vi "ReadSIAM-Ring.vi"() -> ()   [LabVIEW 2011]
panel:
  in  "Motor-Ticket-Konstants":u32[](array[numeric])=[544, 545, 546, 547, 548] format="%.0x"
  in  "ResolutionBits-Table":u8[][](array[numeric])=[[24, 20, 8, 8], [24, 20, 8, 8], [24, 20, 8, 8], [24, 20, 8, 8], [24, 20, 8, 8]]
  in  "Type":u16(ring) items=["acceleration", "velocity", "position", "offset"]
  in  "Motor":T1(ring)
  in  "Tickets":u16(ring) items=["stdout"=512, "framecountdown"=515, "x"=528, "y"=529, "z"=530, "objective-changer"=531, "maindichro"=532, "Trans-motor5"=533, "FRET-motor6"=534, "SI-motor7"=535, "Galvo0"=544, "Galvo1"=545, "x-Galvo"=546, "y-Galvo"=547, "z-TMSI"=548]
  out "Descriptions":cluster{u32, "ValueText":string}[](array[cluster])=[{17305600, "ValueText"="read status of x-motor, 0=ON_AND_NOT_INIT, 1=ON_AND_INIT, 3=offandinit"}, {17760263, "ValueText"="init x-motor, needs some seconds"}, {16781312, "ValueText"="read x-Motor absolute position in uSteps"}, {16777217, "ValueText"="x-Motor write absolute position in uSteps"}, {16842753, "ValueText"="x-Motor write relative position in uSteps"}, {18354176, "ValueText"="read status of y-motor, 0=ON_AND_NOT_INIT, 1=ON_AND_INIT, 3=offandinit"}, {18808839, "ValueText"="init y-motor, needs some seconds"}, {17829888, "ValueText"="read y-Motor absolute position in uSteps"}, {17825793, "ValueText"="y-Motor write absolute position in uSteps"}, {17891329, "ValueText"="y-Motor write relative position in uSteps"}, {19402752, "ValueText"="read status of z-motor, 0=ON_AND_NOT_INIT, 1=ON_AND_INIT, 3=offandinit"}, {19857415, "ValueText"="init z-motor, needs some seconds"}, {19857423, "ValueText"="stop z-motor, go out of closed loop"}, {19857422, "ValueText"="start z-motor, go into closed loop"}, {18878464, "ValueText"="read z-Motor absolute position in uSteps"}, {18874369, "ValueText"="z-Motor write absolute position in uSteps"}, {18939905, "ValueText"="z-Motor write relative position in uSteps"}, {4027514895, "ValueText"="end without ticket"}, {4027518991, "ValueText"="end with ticket"}, {218107904, "ValueText"="IO-read_bank0"}, {218103809, "ValueText"="IO-write_bank0"}, {219156480, "ValueText"="IO-read_bank1"}, {219152385, "ValueText"="IO-write_bank1"}, {218365953, "ValueText"="next bank0 with highres delay no other IO-write until IO done"}, {218365955, "ValueText"="next bank0 with highres delay, value from variable"}, {3289124864, "ValueText"="read background-measured 100MHz ticks between 256 camclocks"}, {3289120770, "ValueText"="store background-measured 100MHz ticks between 256 camclocks to var"}, {3289190400, "ValueText"="read background-measured 100MHz ticks between rizing cam and 10us"}, {3288989697, "ValueText"="set delay in 100MHz ticks to avoid small result, avoid trigger problems, 100"}, {3289055233, "ValueText"="set future 10µs cycels to calculate modulo"}, {3289055235, "ValueText"="set future 10µs cycels from variable# to calculate modulo"}, {3289317386, "ValueText"="do the modulo calculation, after that the result registers are valid"}, {3289251842, "ValueText"="store modulo result in user variable n"}, {4060086278, "ValueText"="ad value to variable"}, {4060090368, "ValueText"="read variable n"}, {4060086273, "ValueText"="set variable n"}, {4060086276, "ValueText"="copy variable m to n"}, {4043374945, "ValueText"="decrement var and branch (0=same line) if equal, I32"}, {4043375201, "ValueText"="decrement var and branch (0=same line) if greater or equal, I32"}, {4043379297, "ValueText"="decrement and branch (0=same line) if greater or equal"}, {4043375457, "ValueText"="decrement and branch (0=same line) if smaller, I32"}, {4043375473, "ValueText"="increment and branch (0=same line) if smaller, I32"}, {102760689, "ValueText"="x-Galvo,data order o,pos,vel,acc"}, {103809265, "ValueText"="y-Galvo,o,pos,vel,acc"}, {104857841, "ValueText"="z-focus,o,pos,vel,acc"}, {102760513, "ValueText"="x-Galvo,pos in data1"}, {103809089, "ValueText"="y-Galvo,pos in data1"}, {104857665, "ValueText"="z-focus,pos in data1"}, {102764609, "ValueText"="x-Galvo,pos in data1, ticket"}, {103813185, "ValueText"="y-Galvo,pos in data1, ticket"}, {104861761, "ValueText"="z-focus,pos in data1, ticket"}, {102764608, "ValueText"="read x-Galvo-pos,ticket"}, {103813184, "ValueText"="read y-Galvo-pos,ticket"}, {104861760, "ValueText"="read z-Focus-pos,ticket"}, {102760515, "ValueText"="set x-Galvo-pos from variable"}, {103809091, "ValueText"="set y-Galvo-pos from variable"}, {104857667, "ValueText"="set z-Focus-pos from variable"}] {"?" format="%.0x"}
  in  "command":u32(ring)=4027514895 format="%x" items=["end_no_ticket"=4027514895, "end_ticket"=4027518991, "NoOp"=4026531840, "Read ticks"=4026535936, "Read ticks to var"=4026535938, "Read IP"=4043313152, "Read IP into var"=4043313154, "Set IP from var"=4043309059, "Set IP from var, relative"=4043313155, "branchRel_if_equal"=4043374849, "decrement_branchRel_if_equal"=4043374945, "decrement_branchRel_if_greaterequal"=4043375201, "decrement_branchRel_if_greaterequal_withTicket"=4043379297, "decrement_branchRel_if_smaller"=4043375457, "increment_branchRel_if_smaller"=4043375473, "readVar"=4060090368, "writeVar"=4060086273, "copyVar0_from_var1"=4060086275, "math_addToVariable"=4076863488, "math_addVToVariable"=4076863489, "math_subToVariable"=4076863490, "math_subVToVariable"=4076863491, "math_multToVariable"=4076863492, "math_multvToVariable"=4076863493, "math_divideToVariable"=4076863494, "math_divideVToVariable"=4076863495, "math_modToVariable"=4076863496, "math_modVToVariable"=4076863497, "logic_and"=4093640704, "logic_or"=4093640706, "logic_xor"=4093640708, "bitshift"=4093640712, "I2C-write"=335544337, "I2C-read"=335548433, "Cam-SPI-write"=3254779905, "UART0-VC-Baud-write"=469958673, "UART0-VC-Baud-read"=469962768, "UART0-VC-write"=469762065, "UART0-VC-write-Var"=469762067, "UART0-VC-read-availabe-bytes-to-var"=470355970, "UART0-VC-read-availabe-bytes"=470355984, "UART0-VC-read-skip-bytes"=469831681, "UART0-VC-read"=469766160, "UART0-VC-read-Var"=469766162, "UART1-TSM-Baud-write"=486735889, "UART1-TSM-Baud-read"=486739984, "UART1-TSM-write"=486539281, "UART1-TSM-write-Var"=486539283, "UART1-TSM-read-availabe-bytes-to-var"=487133186, "UART1-TSM-read-availabe-bytes"=487133200, "UART1-TSM-read-skip-bytes"=486604801, "UART1-TSM-read-skip-bytes"=486608897, "UART1-TSM-read"=486543376, "UART1-TSM-read-Var"=486543378, "UART2-Laser-Baud-write"=503513105, "UART2-Baud-read"=503517200, "UART2-write"=503316497, "UART2-write-Var"=503316499, "UART2-read-availabe-bytes-to-var"=503910402, "UART2-read-availabe-bytes"=503910416, "UART2-read-skip-bytes"=503386113, "UART2-read"=503320592, "UART2-read-Var"=503320594, "UART3-Baud-write"=520290321, "UART3-Baud-read"=520294416, "UART3-write"=520093713, "UART3-write-Var"=520093715, "UART3-read-availabe-bytes-to-var"=520687618, "UART3-read-availabe-bytes"=520687632, "UART3-read-skip-bytes"=520163329, "UART3-read"=520097808, "UART3-read-Var"=520097810, "IO-read_bank0"=3489665024, "IO-write_bank0"=3489660929, "IO-read_bank1"=3506442240, "IO-write_bank1"=3506438145, "DA0-0_LED365"=2684354561, "DA0-1_LED385"=2685403137, "DA0-2_LED440"=2686451713, "DA0-3_LED470"=2687500289, "DA0-4_LED510"=2688548865, "DA0-5_LED550"=2689597441, "DA0-6_LED590"=2690646017, "DA0-7_LED640"=2691694593, "DA1-0_LED-R"=2701131777, "DA1-1_LED-G"=2702180353, "DA1-2_LED-B"=2703228929, "DA1-3_LED-AF"=2704277505, "DA1-4"=2705326081, "DA1-5"=2706374657, "DA1-6"=2707423233, "DA1-7"=2708471809, "DA2-Laser0"=2717908993, "DA2-Laser1"=2718957569, "DA2-Laser2"=2720006145, "DA2-Laser3"=2721054721, "DA2-Laser4"=2722103297, "Analog-read_AD0-0"=2818576384, "Analog-read-store_AD0-0"=2818572290, "AF-Register-transfer r/w"=2835349505, "AF-Register-read"=2835353600, "AF-Register-read-to-var"=2835353602, "AF-Transfer-from-var"=2835349507, "IO-delay_bank0"=3489923073, "IO-delay_bank0_fromVar"=3489923075, "read_cam_clock"=3289124864, "store_cam_clock"=3289120770, "read_cam_phase"=3289190400, "store_cam_phase"=3289186306, "store_cam_phase-t"=3289190402, "r_cam1_NHS"=3254980608, "w_cam1_NHS"=3254976513, "r_cam1_NVS"=3255046144, "w_cam1_NVS"=3255042049, "r_cam1_npx"=3255111680, "w_cam1_npx"=3255107585, "r_cam1_npy"=3255177216, "w_cam1_npy"=3255173121, "r_cam1_xhswait"=3255439360, "w_cam1_xhswait"=3255435265, "r_cam1_xvs_wait"=3255504896, "w_cam1_xvs_wait"=3255500801, "r_cam1_framcounter"=3255570432, "r_cam1_line"=3255635968, "r_cam1_xhs-counter"=3255701504, "r_cam2_NHS"=3271757824, "w_cam2_NHS"=3271753729, "r_cam2_NVS"=3271823360, "w_cam2_NVS"=3271819265, "r_cam2_npx"=3271888896, "w_cam2_npx"=3271884801, "r_cam2_npy"=3271954432, "w_cam2_npy"=3271950337, "r_cam2_xvs_wait"=3272282112, "w_cam2_xvs_wait"=3272278017, "r_cam2_framcounter"=3272347648, "r_cam2_line"=3272413184, "r_cam2_xhs-counter"=3272478720, "start TMSI"=102694919, "set_1Galvo"=101712113, "set_x-Galvo"=102760689, "set_y-Galvo"=103809265, "set_z-Fokus"=104857841, "set_1Galvo_position-only"=101711937, "set_x-Galvo_position-only"=102760513, "set_y-Galvo_position-only"=103809089, "set_z-Fokus_position-only"=104857665, "set_x-Galvo_position-only_ticket"=102764609, "set_y-Galvo_position-only_ticket"=103813185, "set_z-Fokus_position-only_ticket"=104861761, "set_1Galvo_relativ-only"=101712001, "set_x-Galvo_relativ-only"=102760577, "set_y-Galvo_relativ-only"=103809153, "set_z-Fokus_relativ-only"=104857729, "set_1Galvo_speed-only"=101711905, "set_x-Galvo_speed-only"=102760481, "set_y-Galvo_speed-only"=103809057, "set_z-Fokus_speed-only"=104857633, "set_1Galvo_acc-only"=101711889, "set_x-Galvo_acc-only"=102760465, "set_y-Galvo_acc-only"=103809041, "set_z-Fokus_acc-only"=104857617, "read_1Galvo_ticket"=101716032, "read_x-Galvo_ticket"=102764608, "read_y-Galvo_ticket"=103813184, "read_z-Focus_ticket"=104861760, "x-Galvo_pos_fromVar"=102760515, "y-Galvo_pos_fromVar"=103809091, "z-Focus_pos_fromVar"=104857667, "Servo0"=67108865, "Servo0-enable"=68091911, "Servo0-disable"=68091919, "Servo1"=68157441, "Servo1-enable"=69140487, "Servo1-disable"=69140495, "Servo2-enable"=70189063, "Servo2"=69206017, "Servo3-enable"=71237639, "Servo3"=70254593, "x-ssi-init"=202309639, "x-ssi-disable"=202309647, "x-ssi-Bits"=201523201, "x-ssi-Read"=201330688, "x-ssi-ReadToVar"=201326594, "x-ssi-ReadToVar-ticket"=201330690, "y-ssi-init"=203358215, "y-ssi-disable"=203358223, "y-ssi-Bits"=202571777, "y-ssi-Read"=202379264, "y-ssi-ReadToVar"=202375170, "y-ssi-ReadToVat-ticket"=202379266]
  in  "String":string="/* This is a idea of a program readable SAM command description, perhaps we could get that from the board? */\n/* 2021.12.07 new version for ImgProc1-FPGA, rename to RIC!*/\n/* Only the DeviceID+Command and Data structure is explained, communication commands are quite fixed! */\n/* all Values are 32bit, usually signed integer */\n/* there is 8x32bits, a relative time, a command, 5 values (data0 to data4), and data5 for the return ticket */\n/* up to ~14 commands are possible with time delay=0 */\n/* last 4 command bit: 0=read, 1=write, 2=store to var, 3=load from var\" */\n/* xxxx1xxx command ist with ticket return */\n/* TMSI data alignment change after Rev 3 (bug between 3.1-3.8) */\n/* raw commands changed 2018 xxxxxx10, obsolete?, raw read now fpga does not wait */\n/* \\\\till-server\\work\\Projekte allgemein\\Platinen\\SAM-Boards\\SAM2 Board v1.0 Paraxent\\SAM2_Board_all_opcodes.xlsx  */\n\n/*Slow motors via Linux: Does not exist any more; use UART raw! */\n/* fast 10µs commands */\n/*program commands */\ncommand=\"OxF00F000F\" name=\"end_no_ticket\" description=\"end without ticket\"\ncommand=\"OxF00F100F\" name=\"end_ticket\" description=\"end with ticket\" data5-description=\"return-ticket\"\ncommand=\"0xF0000000\" name=\"NoOp\" description=\"Nix, eigentlich...tickcounter\"\n/* 10µs tick counter */\ncommand=\"0xF0001000\" name=\"Read ticks\" description=\"read 10µs counter\"\ncommand=\"0xF0001002\" name=\"Read ticks to var\" description=\"store 10µs to variable\" data0-description=\"variable#\"\n/* Instruction pointer manipulation = jumps */\ncommand=\"0xF1001000\" name=\"Read IP\" description=\"read Instruction pointer\" data5-description=\"return-ticket\"\ncommand=\"0xF1001002\" name=\"Read IP into var\" description=\"read Instruction pointer into variable\" data0-type=U32 data0-description=\"Var#\" data5-description=\"return-ticket\"\ncommand=\"0xF1000003\" name=\"Set IP from var\" description=\"set Instruction pointer from variable\" data0-type=U32 data0-description=\"Var#\"\ncommand=\"0xF1001003\" name=\"Set IP from var, relative\" description=\"set Instruction pointer from variable, relative to actual pointer\" data0-type=U32 data0-description=\"Var# with signed I32\" data5-description=\"return-ticket\"\n/* branch */\ncommand=\"0xF1010101\" name=\"branchRel_if_equal\" description=\"branch (0=same line) if var# equal konstant, I32\" data0-descrition=\"relative jump lines 0=same line\" data0-type=I32 data1-description=\"variable# (0-FF)\" data2-description=\"compare value\" data2-type=I32 \ncommand=\"0xF1010161\" name=\"decrement_branchRel_if_equal\" description=\"decrement var and branch (0=same line) if equal, I32\" data0-descrition=\"relative jump lines 0=same line\" data0-type=I32 data1-description=\"variable# (0-??)\" data2-description=\"compare value\" data2-type=I32 \ncommand=\"0xF1010261\" name=\"decrement_branchRel_if_greaterequal\" description=\"decrement var and branch (0=same line) if greater or equal, I32\" data0-descrition=\"relative jump lines 0=same line\" data0-type=I32 data1-description=\"variable# (0-FF)\" data2-description=\"compare value\" data2-type=I32 \ncommand=\"0xF1011261\" name=\"decrement_branchRel_if_greaterequal_withTicket\" description=\"decrement and branch (0=same line) if greater or equal\" data0-descrition=\"relative jump lines\" data0-type=I32 data1-description=\"variable# (0-FF)\" data2-description=\"compare value\" data1-type=I32 data5-description=\"return-ticket\" \ncommand=\"0xF1010361\" name=\"decrement_branchRel_if_smaller\" description=\"decrement and branch (0=same line) if smaller, I32\" data0-descrition=\"relative jump lines 0=same line\" data0-type=I32 data1-description=\"variable# (0-FF)\" data2-description=\"compare value\" data2-type=I32 \ncommand=\"0xF1010371\" name=\"increment_branchRel_if_smaller\" description=\"increment and branch (0=same line) if smaller, I32\" data0-descrition=\"relative jump lines 0=same line\" data0-type=I32 data1-description=\"variable# (0-FF)\" data2-description=\"compare value\" data2-type=I32 \n/* variables */\ncommand=\"0xF2001000\" name=\"readVar\" description=\"read variable n\" data0-description=\"variable# (0-??), also registers!\" data5-description=\"return-ticket\"\ncommand=\"0xF2000001\" name=\"writeVar\" description=\"set variable n\" data0-description=\"variable# (0-??)\" data1-description=\"value\" data1-type=I32\ncommand=\"0xF2000003\" name=\"copyVar0_from_var1\" description=\"copy var data1 to var data0\" data0-description=\"traget variable# (0-FF)\" data0-type=U8 data1-description=\"source Variable#\" data1-type=U8\n/* math, result always in data0*/\ncommand=\"0xF3000000\" name=\"math_addToVariable\" description=\"add variable0 and value\" data0-description=\"variable#, result\" data1-description=\"valueI32\"\ncommand=\"0xF3000001\" name=\"math_addVToVariable\" description=\"add variable1 to variable0\" data0-description=\"variable#, result\" data1-description=\"variable#\"\ncommand=\"0xF3000002\" name=\"math_subToVariable\" description=\"sub value from variable0\" data0-description=\"variable#, result\" data1-description=\"valueI32\"\ncommand=\"0xF3000003\" name=\"math_subVToVariable\" description=\"sub variable1 from variable0\" data0-description=\"variable0#, result\" data1-description=\"variable1#\"\ncommand=\"0xF3000004\" name=\"math_multToVariable\" description=\"multiply variable with value\" data0-description=\"variable#, result\" data1-description=\"valueI32\"\ncommand=\"0xF3000005\" name=\"math_multvToVariable\" description=\"multiply variable0 with variable1\" data0-description=\"variable0, result#\" data1-description=\"variable1#\"\ncommand=\"0xF3000006\" name=\"math_divideToVariable\" description=\"divide variable0 with value\" data0-description=\"variable#, result\" data1-description=\"valueI32\"\ncommand=\"0xF3000007\" name=\"math_divideVToVariable\" description=\"divide variable1 with variable2\" data0-description=\"variable0#, result\" data1-description=\"variable1#\"\ncommand=\"0xF3000008\" name=\"math_modToVariable\" description=\"integer devision rest variable/value\" data0-description=\"variable#, result\" data1-description=\"valueI32\"\ncommand=\"0xF3000009\" name=\"math_modVToVariable\" description=\"integer devision rest variable0/variable1\" data0-description=\"variable0#, result\" data1-description=\"variable1#\"\n/* logics */\ncommand=\"0xF4000000\" name=\"logic_and\" description=\"variable and value\" data0-description=\"variable#\" data1-description=\"valueI32\"\ncommand=\"0xF4000002\" name=\"logic_or\" description=\"variable or value\" data0-description=\"variable#\" data1-description=\"valueI32\"\ncommand=\"0xF4000004\" name=\"logic_xor\" description=\"variable exclusiveor value\" data0-description=\"variable#\" data1-description=\"valueI32\"\ncommand=\"0xF4000008\" name=\"bitshift\" description=\"shift bits right = devide 2^n, (do left with mult)\" data0-description=\"variable#\" data1-description=\"valueI32 (0-32?)\"\n/*I2C commands */\ncommand=\"0x14000011\" name=\"I2C-write\" description=\"I2C-write\" data0-descrition=AABBCCDD: AA=i2c-addr Tango0x72, CC send bytes, DD response bytes\", data1-description=\"send byts\", data2-description=\"send bytes\", data5-description=\"return ticket\" \ncommand=\"0x14001011\" name=\"I2C-read\" description=\"I2C-read\" data0-descrition=AABBCCDD: AA=i2c-addr Tango0x72, CC send bytes, DD response bytes\", data1-description=\"send byts\", data2-description=\"send bytes\", data5-description=\"return ticket\" \n/*SPI-Camera commands */\ncommand=\"0xC2000001\" name=\"Cam-SPI-write\" description=\"Cam-Write\" data0-descrition=\"0000writebytes(1-F)00\" data1-description=\"data bytes 1,2,3,4\" data2-description=\"data bytes 5,6,7,8\" data3-description=\"data bytes 9,10,11,12\" data4-description=\"data bytes 13,14,15,16\"\n\n/* UART raw commands */\ncommand=\"0x1C030011\" name=\"UART0-VC-Baud-write\" description=\"DCC22-Baud-write\" data0-descrition=\"9600:0xD, 57600: 0x1001, default>115200: 0x1002\" \ncommand=\"0x1C031010\" name=\"UART0-VC-Baud-read\" description=\"DCC22-Baud-read 9600:0xD, 57600: 0x1001, >115200: 0x1002\" \ncommand=\"0x1C000011\" name=\"UART0-VC-write\" description=\"DCC22-write\" data0-descrition=\"0000writebytes(1-F)00\" data1-description=\"data bytes 1,2,3,4\" data2-description=\"data bytes 5,6,7,8\" data3-description=\"data bytes 9,10,11,12\" data4-description=\"data bytes 13,14,15,16\"\ncommand=\"0x1C000013\" name=\"UART0-VC-write-Var\" description=\"DCC22-write from Var\" data0-descrition=\"0000writebytes(1-4)00, big endian\" data1-description=\"var#\"\ncommand=\"0x1C091002\" name=\"UART0-VC-read-availabe-bytes-to-var\" description=\"DCC22-read available bytes, fifo is 1024 long\" data0-descrition=\"var#\" data5-description=\"return ticket\" \ncommand=\"0x1C091010\" name=\"UART0-VC-read-availabe-bytes\" description=\"DCC22-read available bytes, fifo is 1024 long\" data5-description=\"return ticket\" \ncommand=\"0x1C011001\" name=\"UART0-VC-read-skip-bytes\" description=\"DCC22-read-fifo skip bytes\" data0-descrition=\"number of bytes, should not exced available bytes\" data5-description=\"return ticket\" \ncommand=\"0x1C001010\" name=\"UART0-VC-read\" description=\"DCC22-read, big endian packed in U32\" data0-descrition=\"bytes (1-4), FFFFFFFF=all(but ticket not working)\" data5-description=\"return ticket\" \ncommand=\"0x1C001012\" name=\"UART0-VC-read-Var\" description=\"DCC22-read to Var, big endian\" data0-descrition=\"bytes(01-04)\" data1-description=\"var#\" data5-description=\"return ticket\" \ncommand=\"0x1D030011\" name=\"UART1-TSM-Baud-write\" description=\"TSM-Baud-read 9600:0xD, default>57600: 0x1001, 115200: 0x1002\" \ncommand=\"0x1D031010\" name=\"UART1-TSM-Baud-read\" description=\"TSM-Baud-read 9600:0xD, >57600: 0x1001, 115200: 0x1002\" \ncommand=\"0x1D000011\" name=\"UART1-TSM-write\" description=\"TSM-write\" data0-descrition=\"0000writebytes(1-F)00\" data1-description=\"data bytes 1,2,3,4\" data2-description=\"data bytes 5,6,7,8\" data3-description=\"data bytes 9,10,11,12\" data4-description=\"data bytes 13,14,15,16\"\ncommand=\"0x1D000013\" name=\"UART1-TSM-write-Var\" description=\"TSM-write from Var\" data0-descrition=\"0000writebytes(1-4)00, big endian\" data1-description=\"var#\"\ncommand=\"0x1D091002\" name=\"UART1-TSM-read-availabe-bytes-to-var\" description=\"TSM-read available bytes, fifo is 1024 long\" data0-descrition=\"var#\" data5-description=\"return ticket\" \ncommand=\"0x1D091010\" name=\"UART1-TSM-read-availabe-bytes\" description=\"TSM-read available bytes, fifo is 1024 long\" data5-description=\"return ticket\" \ncommand=\"0x1D010001\" name=\"UART1-TSM-read-skip-bytes\" description=\"TSM-read-fifo skip bytes\" data0-descrition=\"number of bytes, should not exced available bytes, gibts nicht bei sam1\"\ncommand=\"0x1D011001\" name=\"UART1-TSM-read-skip-bytes\" description=\"TSM-read-fifo skip bytes\" data0-descrition=\"number of bytes, should not exced available bytes\" data5-description=\"return ticket\" \ncommand=\"0x1D001010\" name=\"UART1-TSM-read\" description=\"TSM-read, big endian packed in U32\" data0-descrition=\"bytes (1-4), FFFFFFFF=all(old? but ticket not working)\" data5-description=\"return ticket\" \ncommand=\"0x1D001012\" name=\"UART1-TSM-read-Var\" description=\"TSM-read to Var, big endian\" data0-descrition=\"bytes(01-04)\" data1-description=\"var#\" data5-description=\"return ticket\" \ncommand=\"0x1E030011\" name=\"UART2-Laser-Baud-write\" description=\"Laser-Baud-write\" data0-descrition=\"9600:0xD, 57600: 0x1001, default >115200: 0x1002\" \ncommand=\"0x1E031010\" name=\"UART2-Baud-read\" description=\"Laser-Baud-read 9600:0xD, 57600: 0x1001, 115200: 0x1002\" \ncommand=\"0x1E000011\" name=\"UART2-write\" description=\"Laser-write\" data0-descrition=\"0000writebytes(1-F)00\" data1-description=\"data bytes 1,2,3,4\" data2-description=\"data bytes 5,6,7,8\" data3-description=\"data bytes 9,10,11,12\" data4-description=\"data bytes 13,14,15,16\"\ncommand=\"0x1E000013\" name=\"UART2-write-Var\" description=\"Laser-write from Var\" data0-descrition=\"0000writebytes(1-4)00, big endian\" data1-description=\"var#\"\ncommand=\"0x1E091002\" name=\"UART2-read-availabe-bytes-to-var\" description=\"Laser-read available bytes, fifo is 1024 long\" data0-descrition=\"var#\" data5-description=\"return ticket\" \ncommand=\"0x1E091010\" name=\"UART2-read-availabe-bytes\" description=\"Laser-read available bytes, fifo is 1024 long\" data5-description=\"return ticket\" \ncommand=\"0x1E011001\" name=\"UART2-read-skip-bytes\" description=\"Laser-read-fifo skip bytes\" data0-descrition=\"number of bytes, should not exced available bytes\" data5-description=\"return ticket\" \ncommand=\"0x1E001010\" name=\"UART2-read\" description=\"Laser-read, big endian packed in U32\" data0-descrition=\"bytes (1-4), FFFFFFFF=all(but ticket not working)\" data5-description=\"return ticket\" \ncommand=\"0x1E001012\" name=\"UART2-read-Var\" description=\"Laser-read to Var, big endian\" data0-descrition=\"bytes(01-04)\" data1-description=\"var#\" data5-description=\"return ticket\" \ncommand=\"0x1F030011\" name=\"UART3-Baud-write\" description=\"UART3 Baud-write\" data0-descrition=\"9600:0xD, 57600: 0x1001, 115200: 0x1002\" \ncommand=\"0x1F031010\" name=\"UART3-Baud-read\" description=\"uart3-Baud-read 9600:0xD, 57600: 0x1001, 115200: 0x1002-default\" \ncommand=\"0x1F000011\" name=\"UART3-write\" description=\"uart3-write\" data0-descrition=\"0000writebytes(1-F)00\" data1-description=\"data bytes 1,2,3,4\" data2-description=\"data bytes 5,6,7,8\" data3-description=\"data bytes 9,10,11,12\" data4-description=\"data bytes 13,14,15,16\"\ncommand=\"0x1F000013\" name=\"UART3-write-Var\" description=\"uart3-write from Var\" data0-descrition=\"0000writebytes(1-4)00, big endian\" data1-description=\"var#\"\ncommand=\"0x1F091002\" name=\"UART3-read-availabe-bytes-to-var\" description=\"uart3-read available bytes, fifo is 1024 long\" data0-descrition=\"var#\" data5-description=\"return ticket\" \ncommand=\"0x1F091010\" name=\"UART3-read-availabe-bytes\" description=\"uart3-read available bytes, fifo is 1024 long\" data5-description=\"return ticket\" \ncommand=\"0x1F011001\" name=\"UART3-read-skip-bytes\" description=\"uart3-read-fifo skip bytes\" data0-descrition=\"number of bytes, should not exced available bytes\" data5-description=\"return ticket\" \ncommand=\"0x1F001010\" name=\"UART3-read\" description=\"uart3-read, big endian packed in U32\" data0-descrition=\"bytes (1-4), FFFFFFFF=all(but ticket not working), Error E7 if not enaugh data\" data5-description=\"return ticket\" \ncommand=\"0x1F001012\" name=\"UART3-read-Var\" description=\"uart3-read to Var, big endian\" data0-descrition=\"bytes(01-04)\" data1-description=\"var#\" data5-description=\"return ticket\" \n/* Digital IO */\ncommand=\"0xD0001000\" name=\"IO-read_bank0\" description=\"IO-read_bank0\" data0-descrition=\"mask-needed,Bit1=cam0ready,Bit4=TSMx,Bit5=TSMy,Bit7(0x80)=Deckel nicht offen\" data5-description=\"return ticket\" \ncommand=\"0xD0000001\" name=\"IO-write_bank0\" description=\"IO-write_bank0\" data0-descrition=\"mask\" data1-description=\"values 0x1=Cam; 0x800=470nmLED; 0x100000=laser0;1F0 0000 all lasers\"\ncommand=\"0xD1001000\" name=\"IO-read_bank1\" description=\"IO-read_bank1\" data0-descrition=\"mask\" data5-description=\"return ticket\" \ncommand=\"0xD1000001\" name=\"IO-write_bank1\" description=\"IO-write_bank1\" data0-descrition=\"mask\" data1-description=\"values \"\n/* Analog Out */\ncommand=\"0xA0000001\" name=\"DA0-0_LED365\" description=\"DA0-0-write 365\" data0-descrition=\"Analog 0-3,3V\" data0-type=U16\ncommand=\"0xA0100001\" name=\"DA0-1_LED385\" description=\"DA0-1-write 385\" data0-descrition=\"Analog 0-3,3V\" data0-type=U16\ncommand=\"0xA0200001\" name=\"DA0-2_LED440\" description=\"DA0-2-write 440\" data0-descrition=\"Analog 0-3,3V\" data0-type=U16\ncommand=\"0xA0300001\" name=\"DA0-3_LED470\" description=\"DA0-3-write 470\" data0-descrition=\"Analog 0-3,3V\" data0-type=U16\ncommand=\"0xA0400001\" name=\"DA0-4_LED510\" description=\"DA0-4-write 510\" data0-descrition=\"Analog 0-3,3V\" data0-type=U16\ncommand=\"0xA0500001\" name=\"DA0-5_LED550\" description=\"DA0-5-write 5xx\" data0-descrition=\"Analog 0-3,3V\" data0-type=U16\ncommand=\"0xA0600001\" name=\"DA0-6_LED590\" description=\"DA0-6-write 590\" data0-descrition=\"Analog 0-3,3V\" data0-type=U16\ncommand=\"0xA0700001\" name=\"DA0-7_LED640\" description=\"DA0-7-write 640\" data0-descrition=\"Analog 0-3,3V\" data0-type=U16\ncommand=\"0xA1000001\" name=\"DA1-0_LED-R\" description=\"DA1-0-write R\" data0-descrition=\"Analog 0-3,3V\" data0-type=U16\ncommand=\"0xA1100001\" name=\"DA1-1_LED-G\" description=\"DA1-1-write\" data0-descrition=\"Analog 0-3,3V\" data0-type=U16\ncommand=\"0xA1200001\" name=\"DA1-2_LED-B\" description=\"DA1-2-write\" data0-descrition=\"Analog 0-3,3V\" data0-type=U16\ncommand=\"0xA1300001\" name=\"DA1-3_LED-AF\" description=\"DA1-3-write\" data0-descrition=\"Analog 0-3,3V\" data0-type=U16\ncommand=\"0xA1400001\" name=\"DA1-4\" description=\"DA1-4-write\" data0-descrition=\"Analog 0-3,3V\" data0-type=U16\ncommand=\"0xA1500001\" name=\"DA1-5\" description=\"DA1-5-write\" data0-descrition=\"Analog 0-3,3V\" data0-type=U16\ncommand=\"0xA1600001\" name=\"DA1-6\" description=\"DA1-6-write\" data0-descrition=\"Analog 0-3,3V\" data0-type=U16\ncommand=\"0xA1700001\" name=\"DA1-7\" description=\"DA1-7-write\" data0-descrition=\"Analog 0-3,3V\" data0-type=U16\ncommand=\"0xA2000001\" name=\"DA2-Laser0\" description=\"DA2-Laser0-405?write\" data0-descrition=\"Analog 0-65535\" data0-type=U16\ncommand=\"0xA2100001\" name=\"DA2-Laser1\" description=\"DA2-Laser1-488?write\" data0-descrition=\"Analog 0-65535\" data0-type=U16\ncommand=\"0xA2200001\" name=\"DA2-Laser2\" description=\"DA2-Laser2-561?write\" data0-descrition=\"Analog 0-65535\" data0-type=U16\ncommand=\"0xA2300001\" name=\"DA2-Laser3\" description=\"DA2-Laser3-640?write\" data0-descrition=\"Analog 0-65535\" data0-type=U16\ncommand=\"0xA2400001\" name=\"DA2-Laser4\" description=\"DA2-Laser4-extra-write\" data0-descrition=\"Analog 0-65535\" data0-type=U16\n/* Analog in, no hardware available */\ncommand=\"0xA8001000\" name=\"Analog-read_AD0-0\" description=\"AD0-0-read\" data5-descrition=\"ticket\"\ncommand=\"0xA8000002\" name=\"Analog-read-store_AD0-0\" description=\"AD0-0-read\" data0-descrition=\"Variable# (0-FF)\" data0-type=U32\n/*Autofocus SPI communication */\ncommand=\"0xA9000001\" name=\"AF-Register-transfer r/w\" description=\"R/W in AF-Register\" data0-descrition=\"6bit Adresse, 1=write 0=read,0, 24bit Wert bei write; diode0-read:C0000000; diode1-read:C4000000, diode15-read:FC000000, \"\ncommand=\"0xA9001000\" name=\"AF-Register-read\" description=\"Read transferred SPI-register, >2µs later\" data5-descrition=\"ticket\"\ncommand=\"0xA9001002\" name=\"AF-Register-read-to-var\" description=\"Read transferred SPI-register to var, >2µs later\" data0-description=\"Variable#\" data5-descrition=\"ticket\"\ncommand=\"0xA9000003\" name=\"AF-Transfer-from-var\" description=\"var to Transfer SPI-register, not tested\" data0-description=\"Variable#, top 6 bit is adress, 1 write... 24bit values\"\n/* extra command for high resolution delay, take care to not use other IO-write on this bank until the delayed IO is done */\ncommand=\"0xD0040001\" name=\"IO-delay_bank0\" description=\"next bank0 with highres delay no other IO-write until IO done\" data0-descrition=\"delay in 100MHz?\"\ncommand=\"0xD0040003\" name=\"IO-delay_bank0_fromVar\" description=\"next bank0 with highres delay 100MHz, value from variable\" data0-descrition=\"variable#\"\n/* external cam-sync, measure clock, measure phase, do modulo (100MHz-base) */\ncommand=\"0xC40C1000\" name=\"read_cam_clock\" description=\"read background-measured 100MHz ticks between 256 camlineclocks\" data5-description=\"return-ticket\"\ncommand=\"0xC40C0002\" name=\"store_cam_clock\" description=\"store background-measured 100MHz ticks between 256 camlineclocks to var\" data0-description=\"variable#\"\ncommand=\"0xC40D1000\" name=\"read_cam_phase\" description=\"read background-measured 100MHz ticks between rizing camline and last 10us\" data5-description=\"return-ticket\"\ncommand=\"0xC40D0002\" name=\"store_cam_phase\" description=\"store background-measured 100MHz ticks between rizing camline and last 10us to var\" data0-description=\"variable#\"\ncommand=\"0xC40D1002\" name=\"store_cam_phase-t\" description=\"store background-measured 100MHz ticks between rizing camline and last 10us to var\" data0-description=\"variable#\" data5-description=\"return-ticket\"\n/* sensovation camera\ncommand=\"0xC2031000\" name=\"r_cam1_NHS\" description=\"John1 NHS default 964\" data5-description=\"return-ticket\"\ncommand=\"0xC2030001\" name=\"w_cam1_NHS\" description=\"John1 NHS default 964\" data1-description=\"HS divider\"\ncommand=\"0xC2041000\" name=\"r_cam1_NVS\" description=\"John1 NVS default 3730\" data5-description=\"return-ticket\"\ncommand=\"0xC2040001\" name=\"w_cam1_NVS\" description=\"John1 NVS default 3730\" data1-description=\"VS divider=lines\"\ncommand=\"0xC2051000\" name=\"r_cam1_npx\" description=\"John1 x-pixel default 5632\" data5-description=\"return-ticket\"\ncommand=\"0xC2050001\" name=\"w_cam1_npx\" description=\"John1 x-pixel default 5632\" data1-description=\"VS divider=lines\"\ncommand=\"0xC2061000\" name=\"r_cam1_npy\" description=\"John1 y-pixel default 3708 beendet DMA!\" data5-description=\"return-ticket\"\ncommand=\"0xC2060001\" name=\"w_cam1_npy\" description=\"John1 y-pixel default 3708 beendet DMA!\" data1-description=\"VS divider=lines\"\ncommand=\"0xC20A1000\" name=\"r_cam1_xhswait\" description=\"John1 xvs_wait default 100\" data5-description=\"return-ticket\"\ncommand=\"0xC20A0001\" name=\"w_cam1_xhswait\" description=\"John1 xvs_wait default 100\" data1-description=\"xhs_wait\"\ncommand=\"0xC20B1000\" name=\"r_cam1_xvs_wait\" description=\"John1 xvs_wait default 10 war mal für cam1 und2\" data5-description=\"return-ticket\"\ncommand=\"0xC20B0001\" name=\"w_cam1_xvs_wait\" description=\"John1 xvs_wait default 10\" data1-description=\"xvs_wait\"\ncommand=\"0xC20C1000\" name=\"r_cam1_framcounter\" description=\"John1 frames cam1\" data5-description=\"return-ticket\"\ncommand=\"0xC20D1000\" name=\"r_cam1_line\" description=\"John1 actual line cam1\" data5-description=\"return-ticket\"\ncommand=\"0xC20E1000\" name=\"r_cam1_xhs-counter\" description=\"John1 INCK cam1\" data5-description=\"return-ticket\"\ncommand=\"0xC3031000\" name=\"r_cam2_NHS\" description=\"John1 NHS default 964\" data5-description=\"return-ticket\"\ncommand=\"0xC3030001\" name=\"w_cam2_NHS\" description=\"John1 NHS default 964\" data1-description=\"HS divider\"\ncommand=\"0xC3041000\" name=\"r_cam2_NVS\" description=\"John1 NVS default 3730\" data5-description=\"return-ticket\"\ncommand=\"0xC3040001\" name=\"w_cam2_NVS\" description=\"John1 NVS default 3730\" data1-description=\"VS divider=lines\"\ncommand=\"0xC3051000\" name=\"r_cam2_npx\" description=\"John1 x-pixel default 5632\" data5-description=\"return-ticket\"\ncommand=\"0xC3050001\" name=\"w_cam2_npx\" description=\"John1 x-pixel default 5632\" data1-description=\"VS divider=lines\"\ncommand=\"0xC3061000\" name=\"r_cam2_npy\" description=\"John1 y-pixel default 3708 beendet DMA!\" data5-description=\"return-ticket\"\ncommand=\"0xC3060001\" name=\"w_cam2_npy\" description=\"John1 y-pixel default 3708 beendet DMA!\" data1-description=\"VS divider=lines\"\ncommand=\"0xC30B1000\" name=\"r_cam2_xvs_wait\" description=\"John1 xvs_wait default 10 war mal für cam1 und2\" data5-description=\"return-ticket\"\ncommand=\"0xC30B0001\" name=\"w_cam2_xvs_wait\" description=\"John1 xvs_wait default 10\" data1-description=\"xvs_wait\"\ncommand=\"0xC30C1000\" name=\"r_cam2_framcounter\" description=\"John1 frames cam2\" data5-description=\"return-ticket\"\ncommand=\"0xC30D1000\" name=\"r_cam2_line\" description=\"John1 actual line cam2\" data5-description=\"return-ticket\"\ncommand=\"0xC30E1000\" name=\"r_cam2_xhs-counter\" description=\"John1 INCK cam2\" data5-description=\"return-ticket\"\n\n/* TMSI-commands */\ncommand=\"0x061F0007\" name=\"start TMSI\" description=\"switch on TMSI, 61-64 possible\" \ncommand=\"0x061000F1\" name=\"set_1Galvo\" description=\"1Galvo,data order o,pos,vel,acc\" data0-description=\"offset\" data1-description=\"pos\" data2-description=\"vel\" data3-description=\"acc\"\ncommand=\"0x062000F1\" name=\"set_x-Galvo\" description=\"x-Galvo,data order o,pos,vel,acc\" data0-description=\"offset\" data1-description=\"pos\" data2-description=\"vel\" data3-description=\"acc\"\ncommand=\"0x063000F1\" name=\"set_y-Galvo\" description=\"y-Galvo,o,pos,vel,acc\" data0-description=\"offset\" data1-description=\"pos\" data2-description=\"vel\" data3-description=\"acc\"\ncommand=\"0x064000F1\" name=\"set_z-Fokus\" description=\"z-focus,o,pos,vel,acc\" data0-description=\"offset\" data1-description=\"pos\" data2-description=\"vel\" data3-description=\"acc\"\ncommand=\"0x06100041\" name=\"set_1Galvo_position-only\" description=\"Wobbel-Galvo,pos in data1 <<16\" data1-description=\"pos\"\ncommand=\"0x06200041\" name=\"set_x-Galvo_position-only\" description=\"x-Galvo,pos in data1 <<16\" data1-description=\"pos\"\ncommand=\"0x06300041\" name=\"set_y-Galvo_position-only\" description=\"y-Galvo,pos in data1 <<16\" data1-description=\"pos\"\ncommand=\"0x06400041\" name=\"set_z-Fokus_position-only\" description=\"z-focus,pos in data1 <<8\" data1-description=\"pos\"\ncommand=\"0x06201041\" name=\"set_x-Galvo_position-only_ticket\" description=\"x-Galvo,pos in data1, ticket\" data1-description=\"pos\" data5-description=\"return-ticket !data0\" data5-type=U32\ncommand=\"0x06301041\" name=\"set_y-Galvo_position-only_ticket\" description=\"y-Galvo,pos in data1, ticket\" data1-description=\"pos\" data5-description=\"return-ticket !data0\" data5-type=U32\ncommand=\"0x06401041\" name=\"set_z-Fokus_position-only_ticket\" description=\"z-focus,pos in data1, ticket\" data1-description=\"pos\" data5-description=\"return-ticket !data0\" data5-type=U32\ncommand=\"0x06100081\" name=\"set_1Galvo_relativ-only\" description=\"1Galvo,relativ in data0 <<16\" data0-description=\"pos\"\ncommand=\"0x06200081\" name=\"set_x-Galvo_relativ-only\" description=\"x-Galvo,relativ in data0 <<16\" data0-description=\"pos\"\ncommand=\"0x06300081\" name=\"set_y-Galvo_relativ-only\" description=\"y-Galvo,relativ in data0 <<16\" data0-description=\"pos\"\ncommand=\"0x06400081\" name=\"set_z-Fokus_relativ-only\" description=\"z-focus,relativ in data0 <<8\" data0-description=\"pos\"\ncommand=\"0x06100021\" name=\"set_1Galvo_speed-only\" description=\"1Galvo,speed in data2 <<28\" data2-description=\"speed\"\ncommand=\"0x06200021\" name=\"set_x-Galvo_speed-only\" description=\"x-Galvo,speed in data2 <<28\" data2-description=\"speed\"\ncommand=\"0x06300021\" name=\"set_y-Galvo_speed-only\" description=\"y-Galvo,speed in data2 <<28\" data2-description=\"speed\"\ncommand=\"0x06400021\" name=\"set_z-Fokus_speed-only\" description=\"z-focus,speed in data2 <<20\" data2-description=\"speed\"\ncommand=\"0x06100011\" name=\"set_1Galvo_acc-only\" description=\"1Glavo,acc in data3 <<32\" data3-description=\"acc\"\ncommand=\"0x06200011\" name=\"set_x-Galvo_acc-only\" description=\"x-Glavo,acc in data3 <<32\" data3-description=\"acc\"\ncommand=\"0x06300011\" name=\"set_y-Galvo_acc-only\" description=\"y-Glavo,acc in data3 <<32\" data3-description=\"acc\"\ncommand=\"0x06400011\" name=\"set_z-Fokus_acc-only\" description=\"z-focus,acc in data3 <<24\" data3-description=\"acc\"\ncommand=\"0x06101040\" name=\"read_1Galvo_ticket\" description=\"read 1Galvo-pos,ticket\" data5-description=\"return-ticket\" data5-type=U32\ncommand=\"0x06201040\" name=\"read_x-Galvo_ticket\" description=\"read x-Galvo-pos,ticket\" data5-description=\"return-ticket\" data5-type=U32\ncommand=\"0x06301040\" name=\"read_y-Galvo_ticket\" description=\"read y-Galvo-pos,ticket\" data5-description=\"return-ticket\" data5-type=U32\ncommand=\"0x06401040\" name=\"read_z-Focus_ticket\" description=\"read z-Focus-pos,ticket\" data5-description=\"return-ticket\" data5-type=U32\ncommand=\"0x06200043\" name=\"x-Galvo_pos_fromVar\" description=\"set x-Galvo-pos from variable\" data0-description=\"variable# (0-FF)\"\ncommand=\"0x06300043\" name=\"y-Galvo_pos_fromVar\" description=\"set y-Galvo-pos from variable\" data0-description=\"variable# (0-FF)\"\ncommand=\"0x06400043\" name=\"z-Focus_pos_fromVar\" description=\"set z-Focus-pos from variable\" data0-description=\"variable# (0-FF)\"\n/*PWM -Servo, Fan */\ncommand=\"0x04000001\" name=\"Servo0\" description=\"Servo0 Main write absolute position 100000-200000, 0=off\" data0-description=\"absolute position\" data0-type=I32\ncommand=\"0x040F0007\" name=\"Servo0-enable\" description=\"Servo0 Main enable\"\ncommand=\"0x040F000F\" name=\"Servo0-disable\" description=\"Servo0 Main disable\"\ncommand=\"0x04100001\" name=\"Servo1\" description=\"Servo1 Fret write absolute position 100000-200000, 0=off\" data0-description=\"absolute position\" data0-type=I32\ncommand=\"0x041F0007\" name=\"Servo1-enable\" description=\"Servo1 Fret enable\"\ncommand=\"0x041F000F\" name=\"Servo1-disable\" description=\"Servo1 Fret disable\"\ncommand=\"0x042F0007\" name=\"Servo2-enable\" description=\"Servo2\"\ncommand=\"0x04200001\" name=\"Servo2\" description=\"Servo2 write absolute position 100000-200000, 0=off\" data0-description=\"absolute position\" data0-type=I32\ncommand=\"0x043F0007\" name=\"Servo3-enable\" description=\"Servo3 enable\"\ncommand=\"0x04300001\" name=\"Servo3\" description=\"Servo3 write absolute position 100000-200000, 0=off\" data0-description=\"absolute position\" data0-type=I32\n/* Encoder SSI-Absolut */\ncommand=\"0x0C0F0007\" name=\"x-ssi-init\" description=\"Enable x position encoder\"\ncommand=\"0x0C0F000F\" name=\"x-ssi-disable\" description=\"Disabale x position encoder\"\ncommand=\"0x0C030001\" name=\"x-ssi-Bits\" description=\"Set xposition encoder bits, default is 20\" data0-description=\"bits (16-32)\"\ncommand=\"0x0C001000\" name=\"x-ssi-Read\" description=\"Read x position encoder\" data5-description=\"return-ticket\"\ncommand=\"0x0C000002\" name=\"x-ssi-ReadToVar\" description=\"Read x position encoder to var\" data0-description=\"variable# (0-FF)\"\ncommand=\"0x0C001002\" name=\"x-ssi-ReadToVar-ticket\" description=\"Read x position encoder to var\" data0-description=\"variable# (0-FF)\"\ncommand=\"0x0C1F0007\" name=\"y-ssi-init\" description=\"Enable y position encoder\"\ncommand=\"0x0C1F000F\" name=\"y-ssi-disable\" description=\"Disabale y position encoder\"\ncommand=\"0x0C130001\" name=\"y-ssi-Bits\" description=\"Set yposition encoder bits, default is 20\" data0-description=\"bits (16-32)\"\ncommand=\"0x0C101000\" name=\"y-ssi-Read\" description=\"Read y position encoder\" data5-description=\"return-ticket\"\ncommand=\"0x0C100002\" name=\"y-ssi-ReadToVar\" description=\"Read y position encoder to var\" data0-description=\"variable# (0-FF)\"\ncommand=\"0x0C101002\" name=\"y-ssi-ReadToVat-ticket\" description=\"Read y position encoder to var\" data0-description=\"variable# (0-FF)\"\n\n/* define TMSI-mask (bit 4..8) up to 4 values can appear in this order (bit8=mask3=data0..bit4=mask0=data3)! Position is sent in the next timeslot, then pos=pos+vel, then vel=vel+acc */\nTMSI-maskbit=\"0\" name=\"acceleration\"\nTMSI-maskbit=\"1\" name=\"velocity\"\nTMSI-maskbit=\"2\" name=\"position\"\nTMSI-maskbit=\"3\" name=\"offset\"\n/* define bits 20..24 TMSI channel-names\" */\nch=\"0\" name=\"galvo0 never used?\"\nch=\"1\" name=\"galvo1\"\nch=\"2\" name=\"x-galvo\"\nch=\"3\" name=\"y-galvo\"\nch=\"4\" name=\"z\"\n\n/* Rev 3.8., internal TMSI-resolution table, bits below 1, ch4 (rufin) is somehow inverted */\nch=\"0\" TMSI-maskbit=\"0\" I32ResolutionBits=\"24\"  /* ch 0 never iin use?*/\nch=\"0\" TMSI-maskbit=\"1\" I32ResolutionBits=\"20\"\nch=\"0\" TMSI-maskbit=\"2\" I32ResolutionBits=\"8\"\nch=\"0\" TMSI-maskbit=\"3\" I32ResolutionBits=\"8\"\nch=\"1\" TMSI-maskbit=\"0\" I32ResolutionBits=\"24\"  /* a */\nch=\"1\" TMSI-maskbit=\"1\" I32ResolutionBits=\"20\"  /* v */\nch=\"1\" TMSI-maskbit=\"2\" I32ResolutionBits=\"8\"  /* x */\nch=\"1\" TMSI-maskbit=\"3\" I32ResolutionBits=\"8\"  /* dx */\nch=\"2\" TMSI-maskbit=\"0\" I32ResolutionBits=\"24\"  \nch=\"2\" TMSI-maskbit=\"1\" I32ResolutionBits=\"20\"\nch=\"2\" TMSI-maskbit=\"2\" I32ResolutionBits=\"8\"\nch=\"2\" TMSI-maskbit=\"3\" I32ResolutionBits=\"8\"\nch=\"3\" TMSI-maskbit=\"0\" I32ResolutionBits=\"24\"  \nch=\"3\" TMSI-maskbit=\"1\" I32ResolutionBits=\"20\"  \nch=\"3\" TMSI-maskbit=\"2\" I32ResolutionBits=\"8\"\nch=\"3\" TMSI-maskbit=\"3\" I32ResolutionBits=\"8\"\nch=\"4\" TMSI-maskbit=\"0\" I32ResolutionBits=\"24\"  /* a */\nch=\"4\" TMSI-maskbit=\"1\" I32ResolutionBits=\"20\"  /* v */\nch=\"4\" TMSI-maskbit=\"2\" I32ResolutionBits=\"8\"   /* x */\nch=\"4\" TMSI-maskbit=\"3\" I32ResolutionBits=\"8\"   /* dx */\n\n/* i2c-registers */\ni2c-addr=\"0x73\", i2c-register\"0x3\", i2c-data=\"0xFC\", descrition=\"init lid-port\"\ni2c-addr=\"0x73\", i2c-register\"0x1\", i2c-data=\"0x1\", descrition=\"reverse/close?\"\ni2c-addr=\"0x73\", i2c-register\"0x1\", i2c-data=\"0x2\", descrition=\"forward/open?\"\ni2c-addr=\"0x73\", i2c-register\"0x1\", i2c-data=\"0x3\", descrition=\"brake\"\ni2c-addr=\"0x73\", i2c-register\"0x0\", descrition=\"read switches\"\n\n\n/* list of control registers from fpga_rw.h */\nregister=\"0\" name=\"status\" comment=\"bit15 protocol running 0x8080, no:0x80\"\nregister=\"6\" name=\"start_address_reg\"\nregister=\"7\" name=\"current_address_reg\"\nregister=\"9\" name=\"current_time_10us_reg\" comment=\"time of protocol\"\nregister=\"21\" name=\"host_timestamp_reg\"\nregister=\"31\" name=\"version_reg\"\nregister=\"23\" name=\"Fehlerregister\"\n\n/* Names for UserVariable 0-n , do fixed loop counters!, math,... */\nvariable=\"1\" name=\"general purpose\"\nvariable=\"2\" name=\"linecountdown\" description=\"set to 0 to stop during this scanned frame\"\nvariable=\"3\" name=\"framecountdown\" description=\"set to 0 to stop sequence after this frame\"\nvariable=\"4\" name=\"z-position\" descrition=\"z-position HW-units, for stack etc\"\nvariable=\"5\" name=\"brightness\"\nvariable=\"10\" name=\"private\"\n\n/* Known tickets */\nTicket=\"0x48\" name=\"spontane rückantwort, lebe noch, kommt alle paar sekunden\"\nTicket=\"0x50\" name=\"Protokoll ende, war auch mal p 0x70\"\nTicket=\"0x70\" name=\"Protokoll ende\"\n\n/* fixed ticket IDs, 0-FF equal to wrapper-command, 100-1FF fixed by Hardware (spontan errors), 200-??? fixed by Software; 1:1 oder 1:n?, konkret z-rs232 und z-TMSI */\nticket=\"0x200\" name=\"stdout\"\nticket=\"0x203\" name=\"framecountdown\" description=\"usually equal to variable #3\"\nticket=\"0x210\" name=\"x\"\nticket=\"0x211\" name=\"y\"\nticket=\"0x212\" name=\"z\"\nticket=\"0x213\" name=\"objective-changer\"\nticket=\"0x214\" name=\"maindichro\"\nticket=\"0x215\" name=\"Trans-motor5\"\nticket=\"0x216\" name=\"FRET-motor6\"\nticket=\"0x217\" name=\"SI-motor7\"\nticket=\"0x220\" name=\"Galvo0\"\nticket=\"0x221\" name=\"Galvo1\"\nticket=\"0x222\" name=\"x-Galvo\"\nticket=\"0x223\" name=\"y-Galvo\"\nticket=\"0x224\" name=\"z-TMSI\"\n\n/* digital bank0 */\nbit=0 name=\"cam0\"\nbit=1 name=\"cam0-ready?\" type=read\nbit=2 name=\"cam1\"\nbit=3 name=\"lid closed? 1=closed\" type=read\nbit=4 name=\"tmsx?\" type=read\nbit=5 name=\"tsmy?\" type=read\nbit=6 name=\"tsm3?\" type=read\nbit=7 name=\"lid open? 0=open\" type=read\nbit=8 name=\"led0-365\"\nbit=9 name=\"led1-385\"\nbit=10 name=\"led2-440\"\nbit=11 name=\"led3-470\"\nbit=12 name=\"led4-510\"\nbit=13 name=\"led5-550\"\nbit=14 name=\"led6-590\"\nbit=15 name=\"led7-640\"\nbit=16 name=\"durchR\"\nbit=17 name=\"durchG\"\nbit=18 name=\"durchB\"\nbit=19 name=\"AF\"\nbit=20 name=\"Laser0\"\nbit=21 name=\"Laser1\"\nbit=22 name=\"Laser2\"\nbit=23 name=\"Laser3\"\nbit=24 name=\"Laser4\"\nbit=25 name=\"Laserext\"\nbit=26 name=\"Lid\"\nbit=27 name=\"SMB1 out?\"\n\n/* motor status, typisch auch für andere module */\n#define AXIS_IS_ON_AND_NOT_INIT    0x40\n#define AXIS_IS_ON_AND_INIT        0x41\n#define AXIS_IS_OFF_AND_NOT_INIT   0x42\n#define AXIS_IS_OFF_AND_INIT       0x43\n#define AXIS_INIT_ONGOING          0x47\n#define AXIS_IS_MOVING             0x4A\n#define AXIS_IS_IN_ERROR_STATE     0x4E\n#define AXIS_IS_IN_UNKNOWN_STATE   0x4F\n/* RAW UART errors */\n#define USART_COMM_ERROR 0x70 (keine Kommunikation möglich)\n#define USART_READ_ERROR 0x71 (Lesen fehlgeschlagen = zu wenige Bytes vor einem Timeout gelesen)\n#define USART_WRITE_ERROR 0x72 (Senden fehlgeschlagen)\n#define USART_MESSAGE_LENGTH_ERROR 0x73 (geforderte Anzahl an Bytes zu groß)\n#define USART_ILLEGAL_MODULE_ERROR 0x74 (nicht implementiertes UART-Modul)\n#define USART_read not available   0xE7 keine uart daten da\n#define wrong_command              0xE1  (z.b. schreibe read only)\n#define CMD_REGISTER_ACCESS_ERROR 0x69 (falsches Register angesprochen)\n\n/*Error Codes copyied from Siam 0.11 source code quite old??\n#define AXIS_COMM_IO_ERROR         0xA1  description=\"Technosoft Axis not responding, no power? no axis 255?\"\n#define AXIS_TIMEOUT_ERROR         0xA2\n#define AXIS_FILE_IO_ERROR         0xA3\n#define AXIS_UNKNOWN_COMMAND       0xA4\n#define AXIS_CMD_SYNTAX_ERROR      0xA5\n#define AXIS_CMD_NOT_FOUND         0xA6 description=\"Technosoft wrong connection, wrong axis_commands.txt?\"\n#define AXIS_RESPONSE_ERROR        0xA7\n#define AXIS_HOME_POS_ERROR        0xA8\n#define AXIS_INIT_ERROR            0xA9\n#define AXIS_NOT_USED              0xAA\n#define AXIS_UNSUPPORTED_TYPE      0xAB\n#define AXIS_RISK_OF_COLLISION     0xAC\n#define AXIS_NOT_INITIALIZED       0xAE\n#define AXIS_FATAL_ERROR           0xAF\n\n#define MAIN_FILE_IO_ERROR             0xA4\n#define MAIN_MESSAGE_ARG_ERROR         0xAA\n#define MAIN_LOGIN_SUCCESSFUL          0xAD\n#define MAIN_LOGIN_INCORRECT           0xAE\n#define MAIN_LOGIN_FAILED              0xAF\n#define MEM_IO_ERROR                   0xB1\n#define MEM_ALIGN_ERROR                0xB2\n#define MEM_MALLOC_ERROR               0xB3\n#define CMD_NOT_SUPPORTED_ERROR        0xC1\n#define CMD_SYNTAX_ERROR               0xC2\n#define CMD_NUM_OF_PARAMS_ERROR        0xC3\n#define CMD_MEM_ACCESS_ERROR           0xC8\n#define CMD_MESSAGE_ARG_ERROR          0xCA\n#define CMD_VAR_ACCESS_ERROR           0xCC\n#define CMD_MODULE_NOT_EXISTING_ERROR  0xCD\n#define CMD_OVERFLOW_ERROR             0xCE\n#define CMD_GENERAL_ERROR              0xCF\n#define SPI_INIT_ERROR                 0xD1\n#define SPI_SEND_ERROR                 0xD2\n#define USART_INIT_ERROR               0xD7\n#define USART_SEND_ERROR               0xD8\n#define I2C_INIT_ERROR                 0xDB\n#define I2C_SEND_ERROR                 0xDC\n#define TCP_ETH_INIT_ERROR             0xE7\n#define TCP_SOCKET_ERROR               0xE1\n#define TCP_SEND_ERROR                 0xE4\n#define TCP_RECV_ERROR                 0xE5\n#define PWR_CIRCUIT_NOT_INIT_ERROR     0xEC\n#define PWR_ILLEGAL_STATE              0xEE\n#define PWR_COMM_ERROR                 0xEF\n#define FPGA_COMM_IO_ERROR             0xF1\n#define FPGA_READ_ERROR                0xF2\n#define FPGA_WRITE_ERROR               0xF3\n#define FPGA_MEM_ACCESS_ERROR          0xF4\n#define FPGA_MEM_ALIGNMENT_ERROR       0xF5\n#define FPGA_ACCESS_OUT_OF_RANGE       0xF6\n#define FPGA_ILLEGAL_VALUE             0xF7\n#define FPGA_NUM_OF_PARAMS_ERROR       0xF8\n#define FPGA_IN_RESET_ERROR            0xF9\n#define FPGA_PROT_RUN_ERROR            0xFA\n#define FPGA_ERROR_ACTIVE              0xFE\n#define GENERAL_ERROR_CODE_CHAR        0xFF\n#define GENERAL_ERROR_CODE_INT         -1  // only works for signed int, also??\n\n\n"
  # "disconnected from type def. \ncopy past to SIAM_command.ctl"
  # "run, replace with enum, copy paste to Typedef"
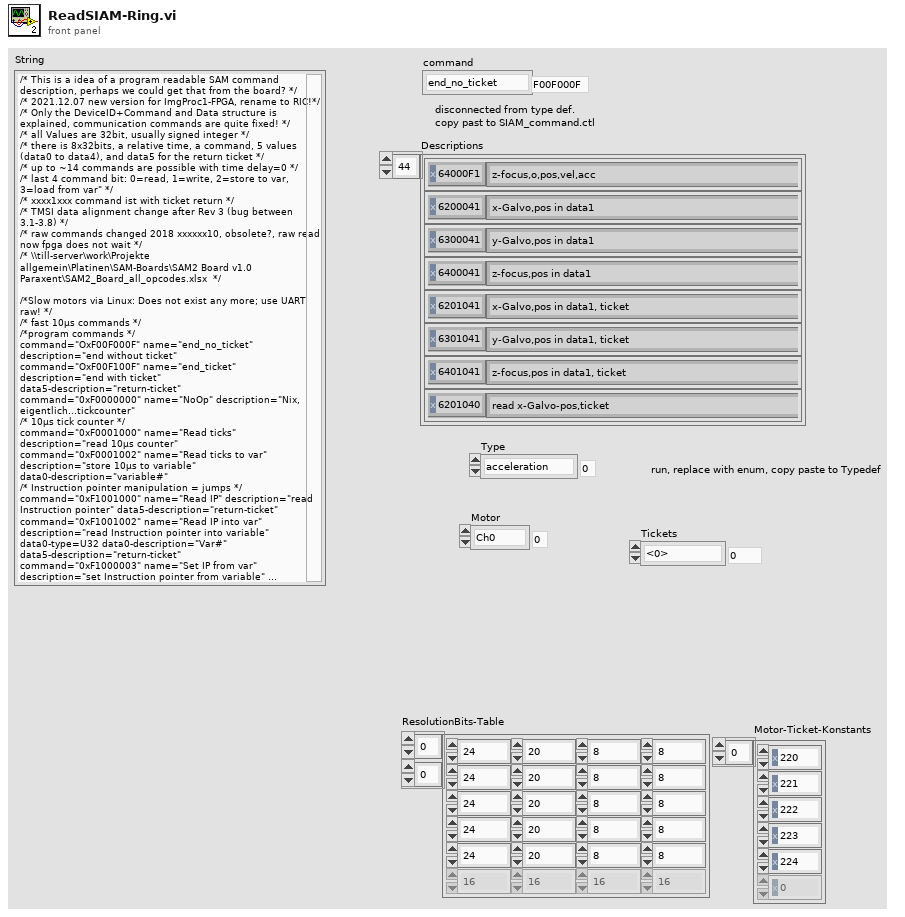
[diagram p1: front panel]
types:
  T1 = enum8{"Ch0", "Ch1", "x-Galvo", "y-Galvo", "z-Focus"}
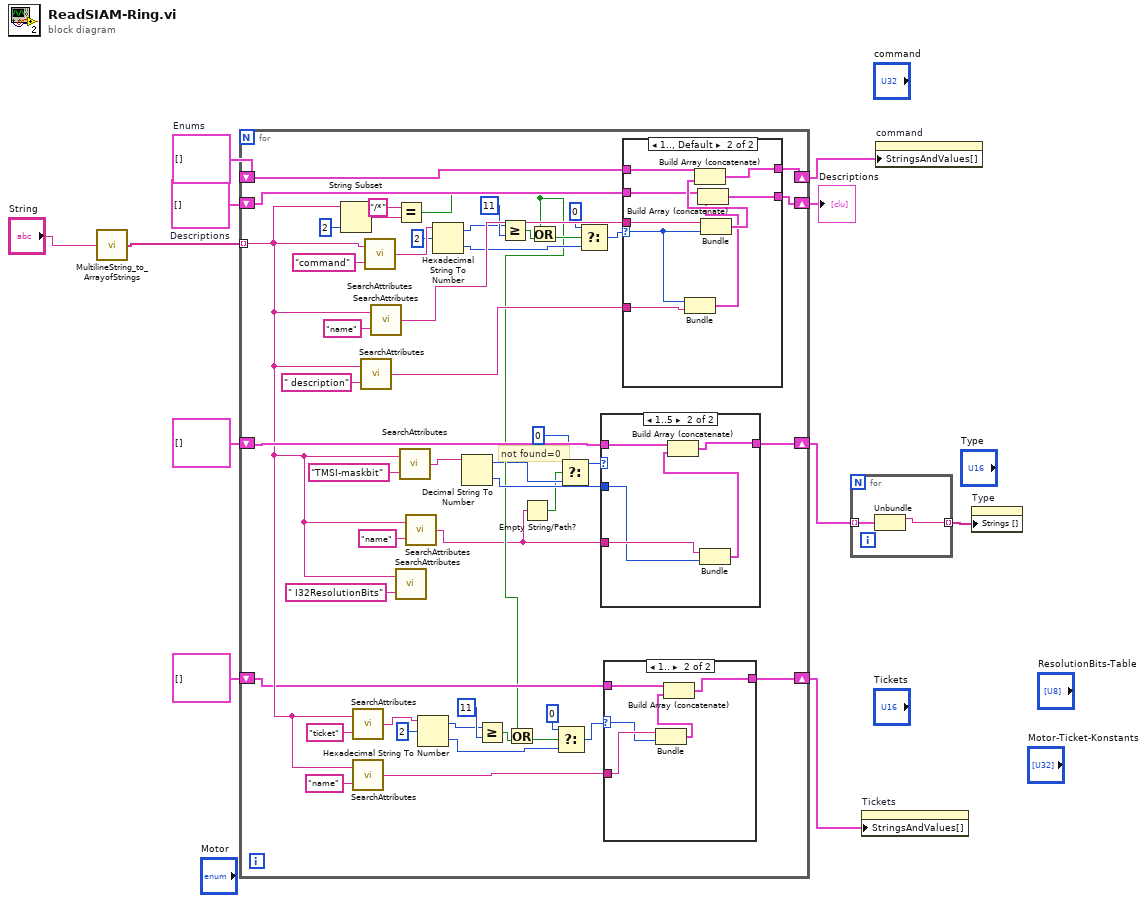
[diagram p0: block diagram]
diagram:
  w7 = cluster{u32, "ValueText":string}[] []  # Descriptions
  w8 = cluster{"ValueText":string, u32}[] []  # Enums
  n1 = call "MultilineString_to_ArrayofStrings.vi"("String 1"="String") -> ("String Array"=w10:string[])  [unwired: 1 in]
  n2 = for {
    tunnel: w10 -> [w30] mode=indexing
    shift-right: [w54] -> w9
    shift-left: w8 -> [w53]
    shift-right: [w46] -> w6
    shift-left: w7 -> [w47]
    shift-right: [w36] -> w2
    shift-left: cluster{"ValueText":string, i32}[] [] -> [w35]
    shift-right: [w26] -> w4
    shift-left: cluster{"ValueText":string, "t":u32}[] [] -> [w27]
    # "not found=0"
    n3 = String Subset(string=w30, length (rest)=2 ("length (rest)")) -> (substring=w43:string)  [unwired: 1 in]
    n4 = call "SearchAttributes.vi"("Search"="ticket", "String"=w30) -> ("ValueText"=w25:string)
    n5 = call "SearchAttributes.vi"("Search"="name", "String"=w30) -> ("ValueText"=w28:string)
    n6 = call "SearchAttributes.vi"("Search"=" description", "String"=w30) -> ("ValueText"=w48:string)
    n7 = call "SearchAttributes.vi"("Search"="command", "String"=w30) -> ("ValueText"=w57:string)
    n8 = call "SearchAttributes.vi"("Search"="name", "String"=w30) -> ("ValueText"=w55:string)
    n9 = Equal?(x="/*", y=w43) -> (x = y?=w17:bool)
    n10 = call "SearchAttributes.vi"("Search"=" I32ResolutionBits", "String"=w30) -> ()  [unwired: 1 out]
    n11 = call "SearchAttributes.vi"("Search"="TMSI-maskbit", "String"=w30) -> ("ValueText"=w34:string)
    n12 = call "SearchAttributes.vi"("Search"="name", "String"=w30) -> ("ValueText"=w16:string)
    n13 = Hexadecimal String To Number(string=w25, offset=2) -> (offset past number=w19:i32, number=w20:u32)  [unwired: 1 in]
    n14 = Hexadecimal String To Number(string=w57, offset=2) -> (offset past number=w45:i32, number=w50:u32)  [unwired: 1 in]
    n15 = Decimal String To Number(string=w34) -> (offset past number=w14:i32, number=w33:i32)  [unwired: 2 in]
    n16 = Greater Or Equal?(x=w19, y=11) -> (x >= y?=w21:bool)
    n17 = Greater Or Equal?(x=w45, y=11) -> (x >= y?=w40:bool)
    n18 = Or(x=w17, y=w21) -> (x .or. y?=w22:bool)
    n19 = Empty String/Path?(string/path=w16) -> (empty?=w13:bool)
    n20 = Or(x=w17, y=w40) -> (x .or. y?=w41:bool)
    n21 = Select(t=u32 0, s=w22, f=w20) -> (s? t:f=w18:u32)
    n22 = Select(t=0, s=w13, f=w14) -> (s? t:f=w15:i32)
    n23 = Select(t=u32 0, s=w41, f=w50) -> (s? t:f=w49:u32)
    n24 = case shown="1..5" w15 {
      tunnel: w33 -> [_ w71]
      tunnel: [w67 w69] -> w36
      tunnel: w35 -> [w67 w70]
      tunnel: w16 -> [_ w72]
      frame 0, Default {
        # "not valid"
      }
      frame 1..5 {
        n25 = Bundle("ValueText"=w72, w71) -> (w68:cluster{"ValueText":string, i32})  [unwired: 1 in]
        n26 = Build Array (concatenate)(w70, w68) -> (w69:cluster{"ValueText":string, i32}[])
      }
    }
    n27 = case shown="1.." w18 {
      selector: w18 -> [_ w62]
      tunnel: w28 -> [_ w66]
      tunnel: w27 -> [w61 w65]
      tunnel: [w61 w64] -> w26
      frame 0, Default {
      }
      frame 1.. {
        n28 = Bundle("ValueText"=w66, "t"=w62) -> (w63:cluster{"ValueText":string, "t":u32})  [unwired: 1 in]
        n29 = Build Array (concatenate)(w65, w63) -> (w64:cluster{"ValueText":string, "t":u32}[])
      }
    }
    n30 = case shown="1.., Default" w49 {
      selector: w49 -> [_ w79]
      tunnel: w55 -> [_ w83]
      tunnel: [w74 w81] -> w54
      tunnel: w53 -> [w74 w80]
      tunnel: w48 -> [_ w78]
      tunnel: w47 -> [w73 w77]
      tunnel: [w73 w76] -> w46
      frame 0 {
        # "not valid"
      }
      frame 1.., Default {
        n31 = Bundle(w79, "ValueText"=w78) -> (w75:cluster{u32, "ValueText":string})  [unwired: 1 in]
        n32 = Build Array (concatenate)(w77, w75) -> (w76:cluster{u32, "ValueText":string}[])
        n33 = Bundle("ValueText"=w83, w79) -> (w82:cluster{"ValueText":string, u32})  [unwired: 1 in]
        n34 = Build Array (concatenate)(w80, w82) -> (w81:cluster{"ValueText":string, u32}[])
      }
    }
  }
  "Descriptions" <- w6
  n35 = for {
    tunnel: w2 -> [w85] mode=indexing
    tunnel: [w84] -> w1 mode=indexing
    n36 = Unbundle(w85) -> ("ValueText"=w84:string)  [unwired: 1 out]
  }
  n37 = property on="Tickets" class="Ring (strict)"("StringsAndValues[]"=w4) -> ()  [unwired: 2 in, 2 out]
  n38 = property on="command" class="Ring (strict)"("StringsAndValues[]"=w9) -> ()  [unwired: 2 in, 2 out]
  n39 = property on="Type" class="Ring (strict)"("Strings []"=w1) -> ()  [unwired: 2 in, 2 out]
